vi "ni579x Read EEPROM.vi"(0 "Register Bus":refnum<class "ni579x Register Bus v1 Host.lvclass">=refnum, 1 "scope":string(combo)="characterization data eeprom", 5 "start address":u32 format="%x", 7 "size":u32, 11 "Error In":errorcluster) -> (4 "Register Bus (out)":refnum<class "ni579x Register Bus v1 Host.lvclass">, 6 "data":u8[](array[numeric]) format="%x", 15 "Error Out":errorcluster)   [LabVIEW 2015]
uses:
  <instrlib>/ni579x/Register Bus/v1/Host/ni579x Register Bus v1 Host.lvclass
  <instrlib>/ni579x/Config/v1/Shared/Types/ni579x FAM Register Offset.ctl
  <instrlib>/ni579x/Config/v1/Shared/Types/ni579x FAM Register Operation.ctl
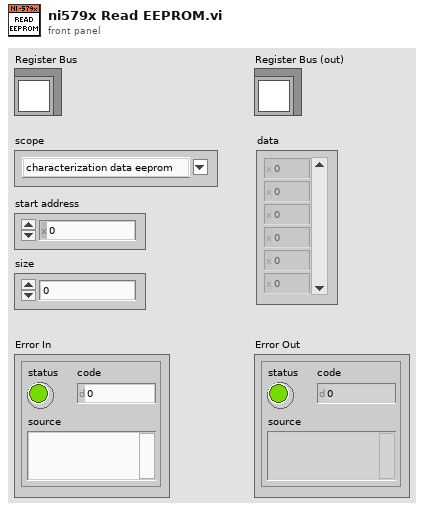
[diagram p1: front panel]
types:
  T1 = typedef "ni579x FAM Register Operation.ctl" = cluster{"FAM Register Offset":T2, "Address":u32, "Write (T)/Read (F)":bool, "Write Data":u32}
  T2 = typedef "ni579x FAM Register Offset.ctl" = u8
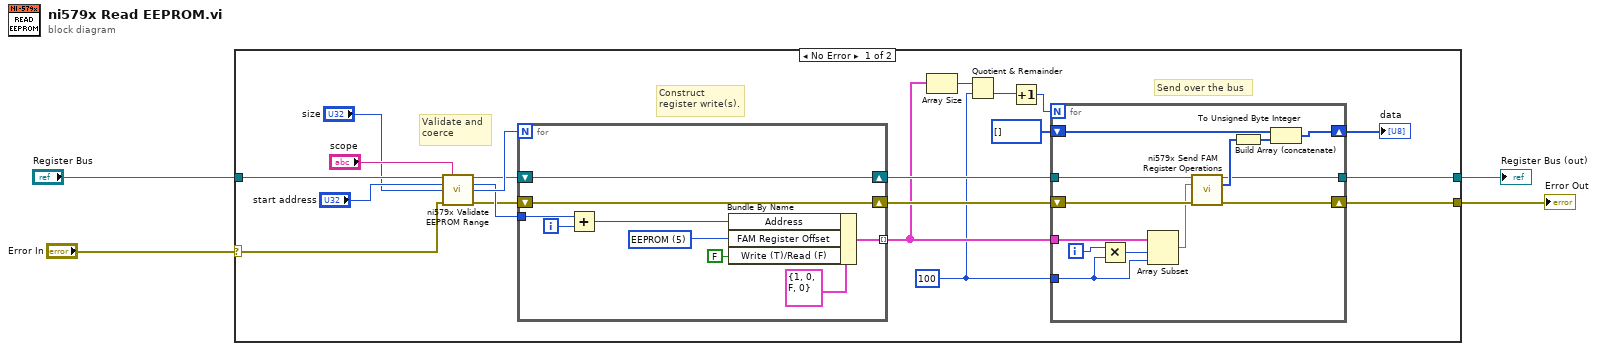
[diagram p0: block diagram]
diagram:
  n1 = case shown="No Error" "Error In" {
    selector: "Error In" -> [w22 w48]
    tunnel: [w12 w48] -> w3
    tunnel: "Register Bus" -> [w24 w47]
    tunnel: [w13 w47] -> w1
    frame No Error {
      w5 = 100 ("length")
      # "Send over the bus"
      # "Construct\nregister write(s)."
      # "Validate and \ncoerce"
      n2 = call <instrlib>:"ni579x Validate EEPROM Range.vi"("Register Bus"=w24, "scope"="scope", "start address"="start address", "size"="size", "Error In"=w22) -> ("Register Bus (out)"=w17:refnum<class "ni579x Register Bus v1 Host.lvclass">, "coerced start address"=w18:u32, "coerced size"=w19:u32, "Error Out"=w16:errorcluster)  [unwired: 7 in]
      n3 = for {
        N: w19 -> [_]
        tunnel: w18 -> [w46]
        shift-right: [w40] -> w14
        shift-left: w16 -> [w40]
        shift-right: [w42] -> w15
        shift-left: w17 -> [w42]
        tunnel: [w41] -> w9 mode=indexing
        i -> [w45]
        w39 = T2 5 items=["ADC"=1, "DAC"=2, "Clock Distribution Chip"=3, "Frequency/Phase Adjust DAC"=4, "EEPROM"=5, "EEPROM Commands"=6, "LO1"=7, "Rx Atten Pre-LNA"=9, "Rx Atten Post-LNA"=10, "Tx Atten"=11] ("FAM Register Offset")
        n4 = Add(x=w46, y=w45) -> (x+y=w43:u32)
        n5 = Bundle By Name(cluster=T1 {"FAM Register Offset"=1, "Address"=0, "Write (T)/Read (F)"=FALSE, "Write Data"=0} ("FAM Register Operation"), "Address"=w43, "FAM Register Offset"=w39, "Write (T)/Read (F)"=FALSE) -> (w41:T1)
      }
      n6 = Array Size(array=w9) -> (size(s)=w8:i32)
      n7 = Quotient & Remainder(x=w8, y=w5) -> (floor(x/y)=w7:i32)  [unwired: 1 out]
      n8 = Increment(x=w7) -> (x+1=w6:i32)
      n9 = for {
        N: w6 -> [_]
        tunnel: w15 -> [w37]
        tunnel: w9 -> [w32]
        tunnel: [w34] -> w13
        shift-right: [w26] -> w10
        shift-left: u8[] [] -> [w27]
        shift-right: [w33] -> w12
        shift-left: w14 -> [w36]
        tunnel: w5 -> [w25]
        i -> [w31]
        n10 = Multiply(x=w31, y=w25) -> (x*y=w30:i32)
        n11 = Array Subset(array=w32, index=w30, length=w25) -> (w29:T1[])
        n12 = call <instrlib>:"ni579x Send FAM Register Operations.vi"("Register Bus"=w37, "FAM Register Operations"=w29, "Error In"=w36) -> ("Register Bus (out)"=w34:refnum<class "ni579x Register Bus v1 Host.lvclass">, "FAM Register Read Data"=w35:u32[], "Error Out"=w33:errorcluster)  [unwired: 10 in]
        n13 = To Unsigned Byte Integer(number=w35) -> (unsigned 8bit integer=w28:u8[])
        n14 = Build Array (concatenate)(w27, w28) -> (w26:u8[])
      }
      "data" <- w10
    }
    frame Error {
    }
  }
  "Register Bus (out)" <- w1
  "Error Out" <- w3
